vi "Generate Memory Allocation.vi"(8 "error in":errorcluster, 11 "Shared Memory configuration in":refnum<class "Shared Memory configuration.lvclass">) -> (0 "error out":errorcluster, 2 "Memory Allocations":T1[](array[typedef]), 3 "Shared Memory configuration out":refnum<class "Shared Memory configuration.lvclass">)   [LabVIEW 2014, in "Shared Memory configuration.lvclass"]
uses:
  Shared Memory configuration.lvclass
  Memory Allocation.ctl
  Line.ctl
  <vilib>/NI/Tag Bus Module Framework/channel/TBM channel.lvclass
  Shared Memory configuration.lvclass/Shared Memory configuration.ctl
  Read Input File String.vi
  Read Output File String.vi
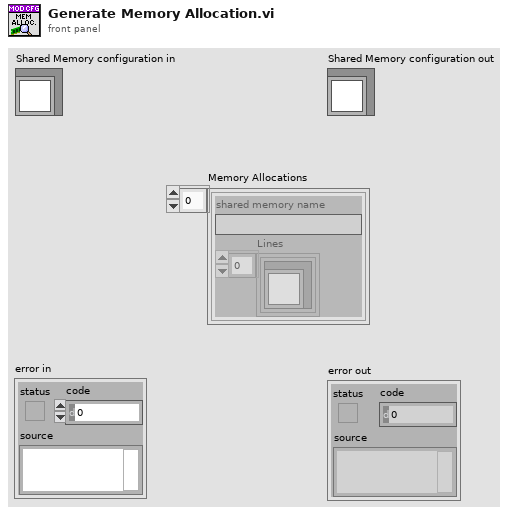
[diagram p1: front panel]
types:
  T1 = typedef "Shared Memory configuration.lvclass/Memory Allocation.ctl" = cluster{"shared memory name":string, "Lines":T2[]}
  T2 = typedef "Shared Memory configuration.lvclass/Line.ctl" = cluster{"channel":refnum<class "TBM channel.lvclass">}
  T3 = typedef "tag bus.lvlib/tag descriptor.lvclass/Data Type.ctl" = enum16{"Double", "Single", "I64", "I32", "I16", "I8", "U64", "U32", "U16", "U8", "Boolean", "String", "Array of Double", "Array of Single", "Array of I64", "Array of I32", "Array of I16", "Array of I8", "Array of U64", "Array of U32", "Array of U16", "Array of U8", "Array of Boolean", "Array of String"}
  T4 = typedef "TBM channel.lvclass/channel classification.ctl" = enum16{"input data", "output data", "processing parameter", "processing result"}
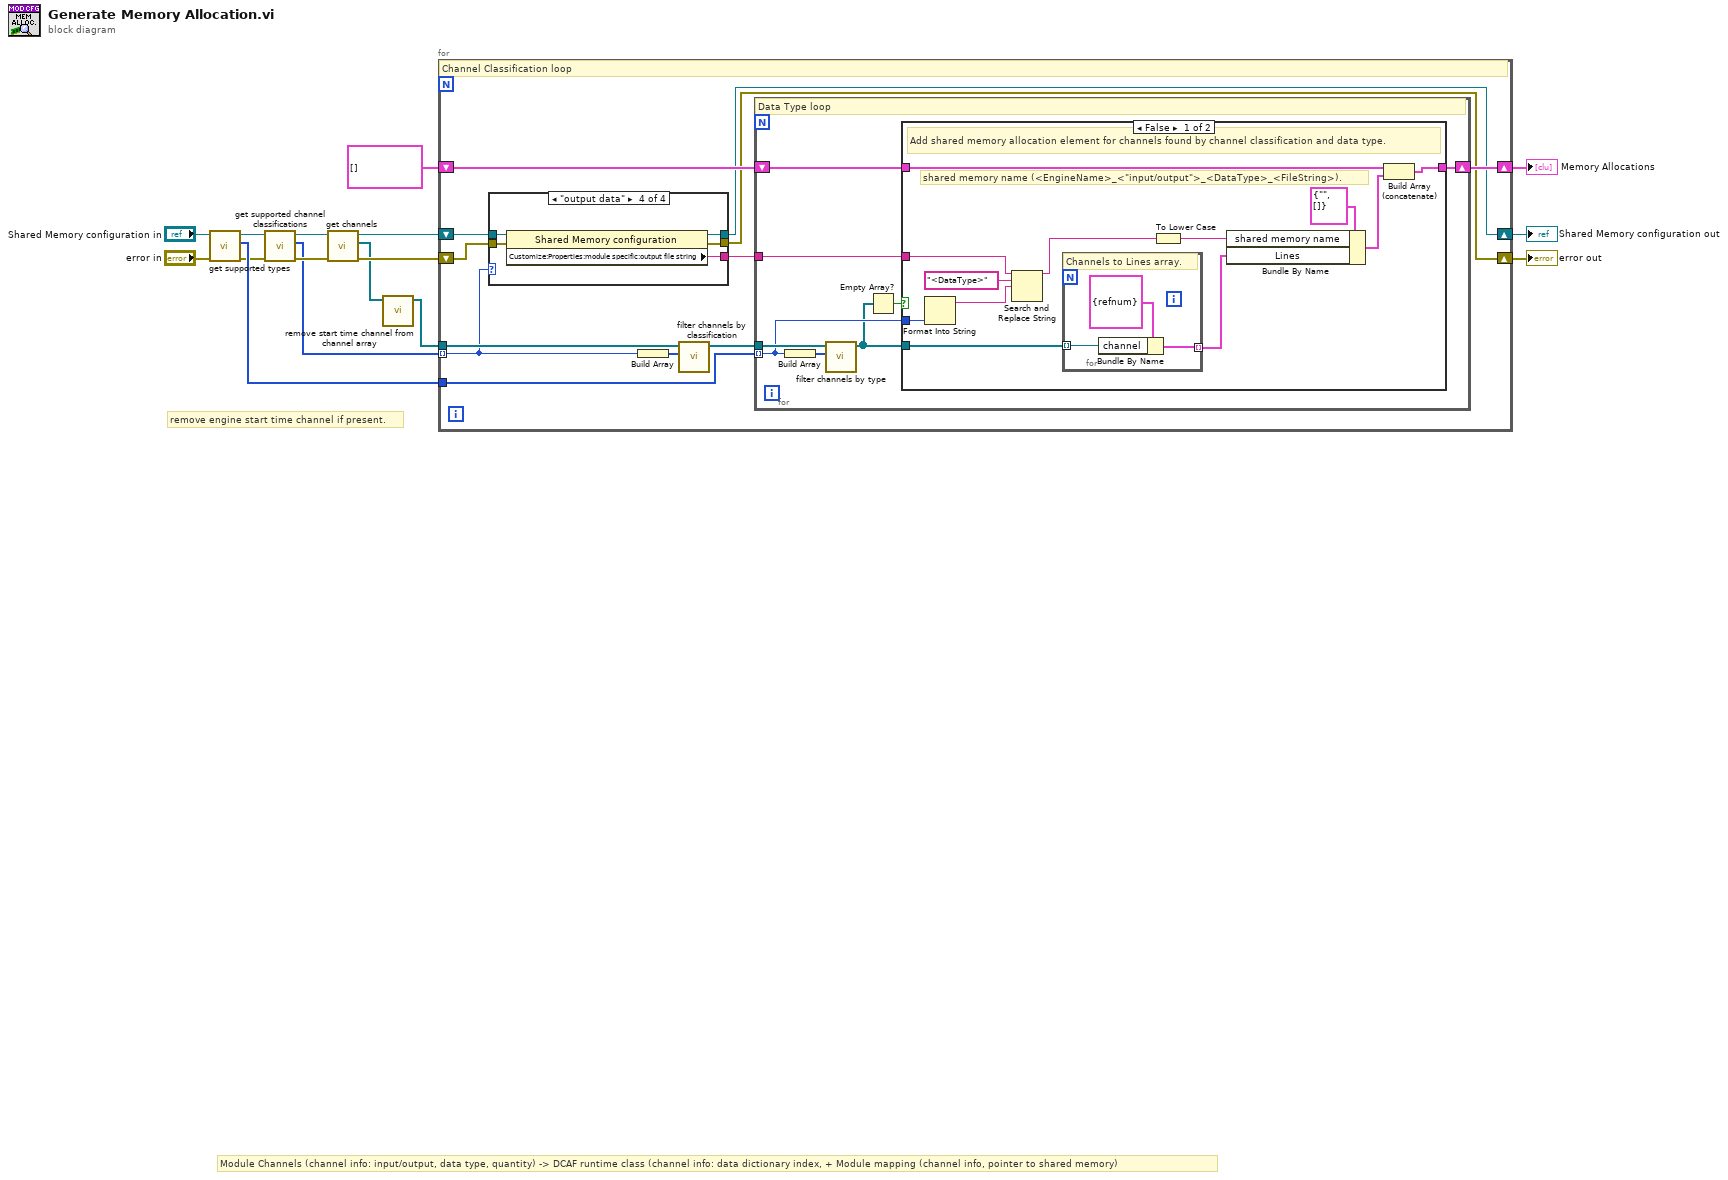
[diagram p0: block diagram]
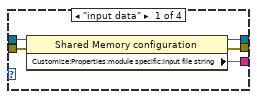
[diagram p3: hidden frame]
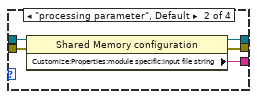
[diagram p4: hidden frame]
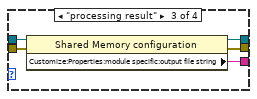
[diagram p5: hidden frame]
diagram:
  # "remove engine start time channel if present."
  # "Module Channels (channel info: input/output, data type, quantity) -> DCAF runtime class (channel info: data dictionary index, + Module mapping (channel info, pointer to shared memory)"
  n1 = call-dynamic "get supported types.vi"("error in"="error in", "Shared Memory configuration in"="Shared Memory configuration in") -> ("error out"=w9:errorcluster, "supported types"=w11:T3[], "Shared Memory configuration out"=w10:refnum<class "Shared Memory configuration.lvclass">)  [unwired: 7 in]
  n2 = call-dynamic "get supported channel classifications.vi"("error in"=w9, "module configuration in"=w10) -> ("error out"=w7:errorcluster, "supported classes"=w2:T4[], "module configuration out"=w5:refnum<class "Shared Memory configuration.lvclass">)  [unwired: 7 in]
  n3 = call-dynamic "get channels.vi"("Shared Memory configuration in"=w5) -> ("channels"=w1:refnum<class "TBM channel.lvclass">[], "Shared Memory configuration out"=w4:refnum<class "Shared Memory configuration.lvclass">)  [unwired: 9 in]
  n4 = call "remove start time channel from channel array.vi"("channels in"=w1) -> ("channels out"=w3:refnum<class "TBM channel.lvclass">[])  [unwired: 10 in]
  n5 = for {
    tunnel: w2 -> [w23] mode=indexing
    shift-right: [w19] -> w14
    shift-left: w4 -> [w22]
    shift-right: [w25] -> w12
    shift-left: T1[] [] -> [w26]
    shift-right: [w20] -> w13
    shift-left: w7 -> [w21]
    tunnel: w11 -> [w27]
    tunnel: w3 -> [w24]
    # "Channel Classification loop"
    n6 = case shown="\"output data\"" w23 {
      tunnel: w22 -> [w56 w61 w66 w71]
      tunnel: w21 -> [w55 w60 w65 w70]
      tunnel: [w52 w59 w62 w67] -> w18
      tunnel: [w54 w58 w64 w69] -> w19
      tunnel: [w53 w57 w63 w68] -> w20
      frame "input data" {
        n7 = property class="Shared Memory configuration"(reference=w56, error in=w55) -> (reference out=w54:refnum<class "Shared Memory configuration.lvclass">, error out=w53:errorcluster, "Customize:Properties:module specific:input file string"=w52:string)
      }
      frame "processing parameter", Default {
        n8 = property class="Shared Memory configuration"(reference=w61, error in=w60) -> (reference out=w58:refnum<class "Shared Memory configuration.lvclass">, error out=w57:errorcluster, "Customize:Properties:module specific:input file string"=w59:string)
      }
      frame "processing result" {
        n9 = property class="Shared Memory configuration"(reference=w66, error in=w65) -> (reference out=w64:refnum<class "Shared Memory configuration.lvclass">, error out=w63:errorcluster, "Customize:Properties:module specific:output file string"=w62:string)
      }
      frame "output data" {
        n10 = property class="Shared Memory configuration"(reference=w71, error in=w70) -> (reference out=w69:refnum<class "Shared Memory configuration.lvclass">, error out=w68:errorcluster, "Customize:Properties:module specific:output file string"=w67:string)
      }
    }
    n11 = Build Array(w23) -> (w17:T4[])
    n12 = call <vilib>:"filter channels by classification.vi"("allowed classifications"=w17, "channels in"=w24) -> ("channels out"=w16:refnum<class "TBM channel.lvclass">[])  [unwired: 9 in]
    n13 = for {
      tunnel: w27 -> [w30] mode=indexing
      tunnel: w18 -> [w33]
      tunnel: w16 -> [w31]
      shift-right: [w34] -> w25
      shift-left: w26 -> [w35]
      # "Data Type loop"
      n14 = Build Array(w30) -> (w32:T3[])
      n15 = call <vilib>:"filter channels by type.vi"("allowed types"=w32, "channels in"=w31) -> ("channels out"=w29:refnum<class "TBM channel.lvclass">[])  [unwired: 9 in]
      n16 = Empty Array?(array=w29) -> (empty?=w28:bool)
      n17 = case shown="False" w28 {
        tunnel: w35 -> [w44 w51]
        tunnel: w29 -> [w46 _]
        tunnel: [w43 w51] -> w34
        tunnel: w30 -> [w39 _]
        tunnel: w33 -> [w38 _]
        frame False {
          # "shared memory name (<EngineName>_<\"input/output\">_<DataType>_<FileString>)."
          # "Add shared memory allocation element for channels found by channel classification and data type."
          n18 = Format Into String(w39) -> (resulting string=w41:string)  [unwired: 3 in, 1 out]
          n19 = Search and Replace String(input string=w38, search string="<DataType>" ("shared memory name"), replace string=w41) -> (result string=w37:string)  [unwired: 5 in, 3 out]
          n20 = for {
            tunnel: w46 -> [w48] mode=indexing
            tunnel: [w49] -> w45 mode=indexing
            # "Channels to Lines array."
            n21 = Bundle By Name(cluster=T2 {"channel"=refnum} ("Line"), "channel"=w48) -> (w49:T2)
          }
          n22 = To Lower Case(string=w37) -> (all lower case string=w36:string)
          n23 = Bundle By Name(cluster=T1 {"shared memory name"="", "Lines"=[]} ("memory allocation"), "shared memory name"=w36, "Lines"=w45) -> (w42:T1)
          n24 = Build Array (concatenate)(w44, w42) -> (w43:T1[])
        }
        frame True {
        }
      }
    }
  }
  "error out" <- w13
  "Shared Memory configuration out" <- w14
  "Memory Allocations" <- w12
